vi "download-files.vi"(8 "error in":errorcluster, 9 "download folder":path, 10 "file list":T1[](array[typedef]), 11 "session handle in":T2) -> (0 "error cout":errorcluster, 3 "session handle out":T2)   [LabVIEW 2020]
uses:
  <vilib>/WebDAVClient/NI_WebDAV.lvlib
  <vilib>/WebDAVClient/Advanced/Get File.vi
  <vilib>/WebDAVClient/Advanced/SessionHandle.ctl
  <vilib>/WebDAVClient/Advanced/FileInfo.ctl
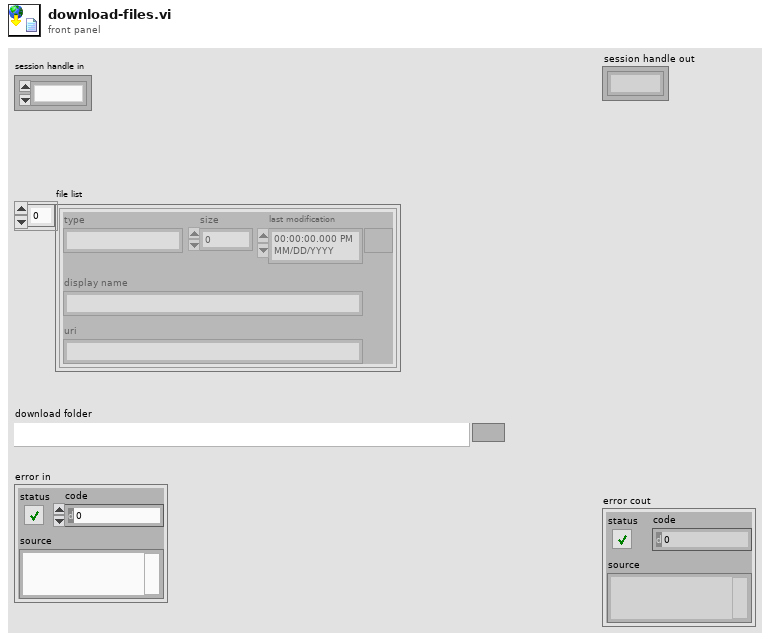
[diagram p1: front panel]
types:
  T1 = typedef "NI_WebDAV.lvlib/FileInfo.ctl" = cluster{"type":string, "size":u64, "last modification":timestamp, "display name":string, "uri":string}
  T2 = typedef "NI_WebDAV.lvlib/SessionHandle.ctl" = refnum<k1>
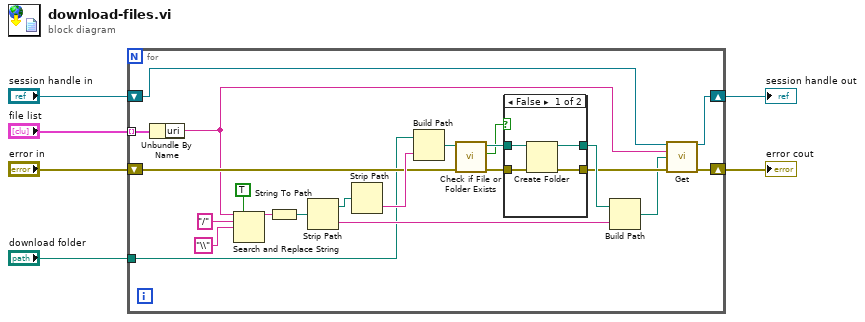
[diagram p0: block diagram]
diagram:
  n1 = for {
    tunnel: "file list" -> [w28] mode=indexing
    shift-right: [w10] -> w1
    shift-left: "error in" -> [w9]
    tunnel: "download folder" -> [w8]
    shift-right: [w11] -> w5
    shift-left: "session handle in" -> [w12]
    n2 = Unbundle By Name(w28) -> ("uri"=w7:string)
    n3 = Search and Replace String(replace all?=TRUE ("replace all? (F)"), input string=w7, search string="/", replace string="\\" ("replace string (\"\")")) -> (result string=w26:string)  [unwired: 4 in, 3 out]
    n4 = String To Path(string=w26) -> (path=w27:path)
    n5 = Strip Path(path=w27) -> (stripped path=w22:path, name=w15:string)
    n6 = Strip Path(path=w22) -> (name=w16:string)  [unwired: 1 out]
    n7 = Build Path(base path=w8, name or relative path=w16) -> (appended path=w21:path)
    n8 = call <vilib>:"Check if File or Folder Exists.vi"("error in (no error)"=w9, "path"=w21) -> ("error out"=w18:errorcluster, "file or folder exists?"=w19:bool, "dup path"=w20:path)  [unwired: 7 in]
    n9 = case shown="False" w19 {
      tunnel: w20 -> [w32 w33]
      tunnel: w18 -> [w31 w34]
      tunnel: [w30 w34] -> w14
      tunnel: [w29 w33] -> w17
      frame False {
        n10 = Create Folder(path (use dialog)=w32, error in=w31) -> (created path=w29:path, error out=w30:errorcluster)  [unwired: 1 in, 1 out]
      }
      frame True {
      }
    }
    n11 = Build Path(base path=w17, name or relative path=w15) -> (appended path=w13:path)
    n12 = call-poly <vilib>:"Get.vi"("session handle"=w12, "relative uri"=w7, "local file path"=w13, "error in (no error)"=w14) -> ("session handle out"=w11:T2, "error out"=w10:errorcluster)  [unwired: 9 in, 1 out]
  }
  "session handle out" <- w5
  "error cout" <- w1
